vi "Load Firmware ReadMe.vi"(8 "Error In":errorcluster, 9 "Device Family":u16(ring) items=["National Instruments", "Digilent", "Arduino"], 10 "Device Type":u16(ring) items=["chipKIT Uno32", "chipKIT uC32", "chipKIT Max32", "chipKIT DP32"], 11 "Firmware Version":u16(ring) items=["LINX -  Serial / USB", "LINX -  Serial / USB [Debug] "]) -> (0 "Error Out":errorcluster, 3 "Firmware ReadMe":string)   [LabVIEW 2011, in "LVH-LINX.lvlib"]
doc: "Load specified firmware readme."
uses:
  LVH-LINX.lvlib
  Program Files (x86)/LabVIEW Hacker/Build Tools/common/LVH-SystemTools.lvlib
panel:
  in  "Device Family":u16(ring) items=["National Instruments", "Digilent", "Arduino"]
  in  "Device Type":u16(ring) items=["chipKIT Uno32", "chipKIT uC32", "chipKIT Max32", "chipKIT DP32"]
  in  "Firmware Version":u16(ring) items=["LINX -  Serial / USB", "LINX -  Serial / USB [Debug] "]
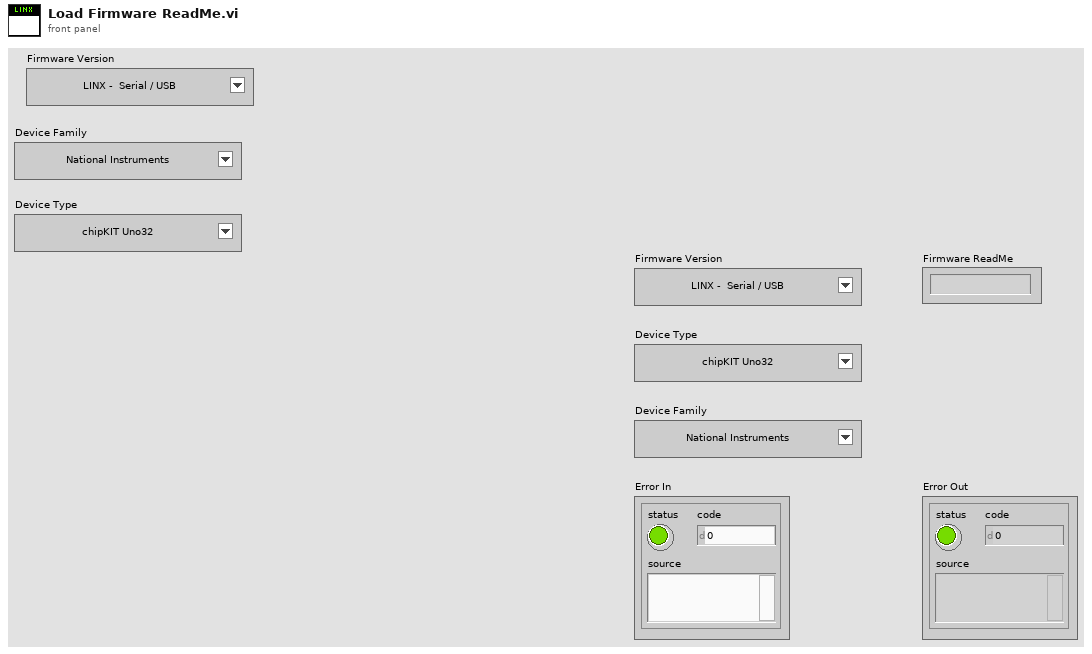
[diagram p1: front panel]
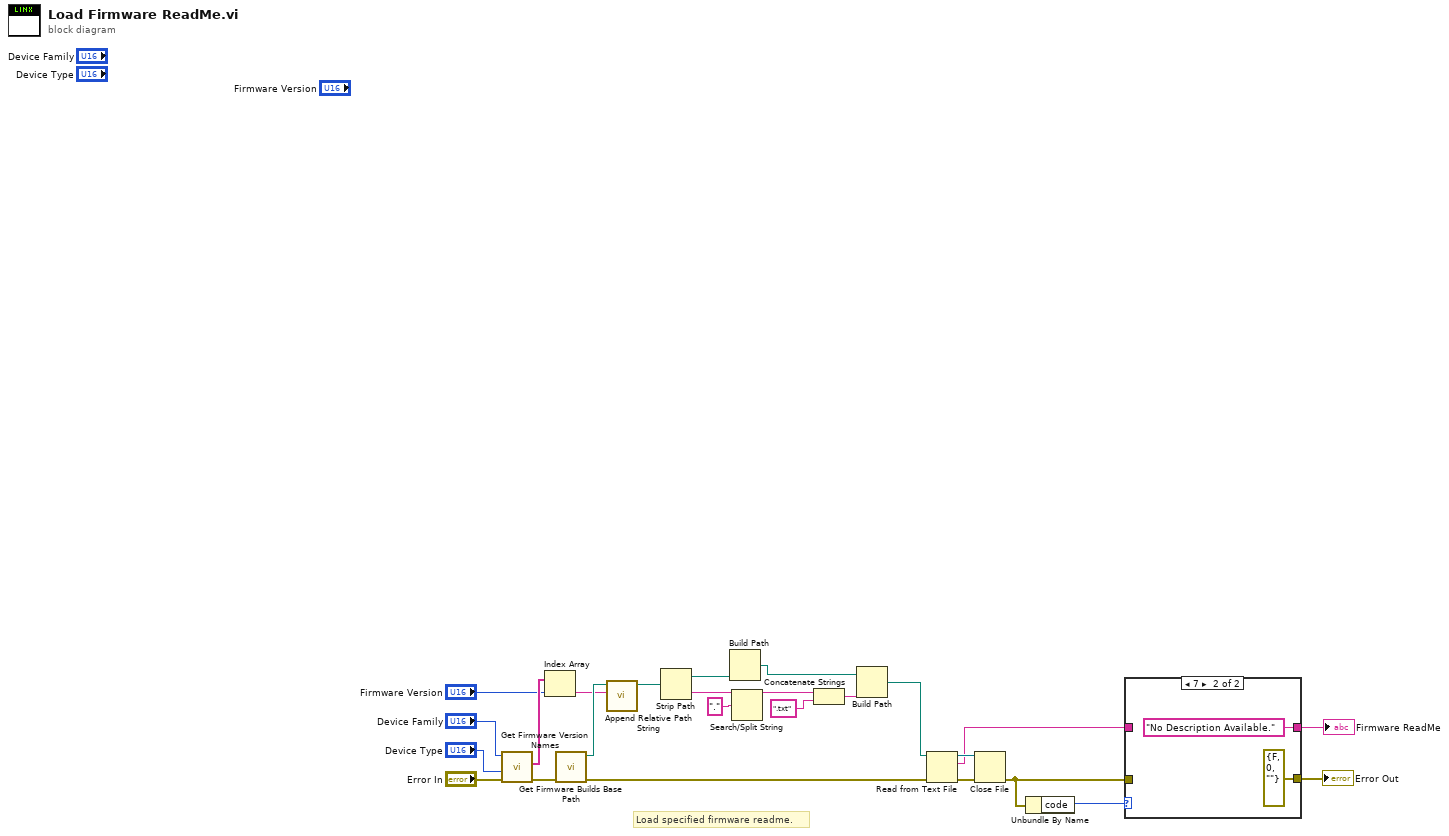
[diagram p0: block diagram]
diagram:
  # "Load specified firmware readme."
  n1 = call "Get Firmware Version Names.vi"("Error In"="Error In", "Device ID"="Device Type", "Device Family"="Device Family") -> ("Error Out"=w24:errorcluster, "Firmware Version Relative Path"=w25:string[])  [unwired: 6 in, 1 out]
  n2 = Index Array(array=w25, index="Firmware Version") -> (element=w22:string)
  n3 = call "Get Firmware Builds Base Path.vi"("Error In"=w24) -> ("Error Out"=w7:errorcluster, "Firmware Builds Base Path"=w23:path)  [unwired: 9 in]
  n4 = call <vilib>:"Append Relative Path String.vi"("Relative Path"=w22, "Base Path"=w23) -> ("Absolute Path"=w14:path)  [unwired: 9 in]
  n5 = Strip Path(path=w14) -> (stripped path=w17:path, name=w21:string)
  n6 = Build Path(name or relative path=w17) -> (appended path=w16:path)  [unwired: 1 in]
  n7 = Search/Split String(string=w21, search string/char (-)=".") -> (substring before match=w19:string)  [unwired: 1 in, 2 out]
  n8 = Concatenate Strings(w19, ".txt" ("string")) -> (w15:string)
  n9 = Build Path(base path=w16, name or relative path=w15) -> (appended path=w8:path)
  n10 = Read from Text File(file (use dialog)=w8, error in=w7) -> (refnum out=w9:refnum<file>, text=w1:string, error out=w10:errorcluster)  [unwired: 2 in, 1 out]
  n11 = Close File(refnum=w9, error in=w10) -> (error out=w4:errorcluster)  [unwired: 1 out]
  n12 = Unbundle By Name(w4) -> ("code"=w5:i32)
  n13 = case shown="7" w5 {
    tunnel: w4 -> [w26 _]
    tunnel: [w26 errorcluster {"status"=FALSE, "code"=0, "source"=""} ("error out")] -> w3
    tunnel: [w27 "No Description Available."] -> w2
    tunnel: w1 -> [w27 _]
    frame 0, Default {
    }
    frame 7 {
    }
  }
  "Error Out" <- w3
  "Firmware ReadMe" <- w2
